vi "Robot Global Data.vi"() -> ()   [LabVIEW 2020]
doc: "This global VI can contain as many global variables as you need. To create a global variable, place a control on the panel, give it a good name. To read or write to it from a VI, drag the icon to the diagram of that VI. You can also drag from the project. Click on the node to change which global you access. You shouldn't have multiple locations writing to a global or it will cause a race-condition."
uses:
  <vilib>/Rock Robotics/WPI/Camera/WPI_CameraImageSize.ctl
  <vilib>/Rock Robotics/WPI/DriverStation/WPI_DriverStationRobotMode2.ctl
  Support Code/submodules/bordeaux-pathinator/Bordeaux/Types/Single Cmd Info.ctl
  <vilib>/picture/picture.llb/imagedata.ctl
  Support Code/submodules/bordeaux-pathinator/Bordeaux/Types/Trajectory Data.ctl
  Support Code/submodules/bordeaux-pathinator/Bordeaux/Types/Segment Type.ctl
  Support Code/submodules/bordeaux-pathinator/Bordeaux/Types/Overrides.ctl
  Support Code/submodules/bordeaux-pathinator/Bordeaux/Types/Angluar Limits.ctl
  Support Code/submodules/bordeaux-pathinator/Bordeaux/Types/Drive Type.ctl
  Support Code/submodules/bordeaux-pathinator/Bordeaux/Types/Path Type.ctl
  Support Code/submodules/numlock/src/numlock.ctl
panel:
  out "Shooter Ready?":bool
  in  "Deadman Switch Active":bool
  out "Climb Sequence Finished":bool
  out "logger":T1
  out "Autos":T10(array[cluster]) {"Fields"."Overrides"."Angle Override" step=5.0; "Fields"."Overrides"."Velocity Override" step=5.0; "Fields"."Overrides"."Angular Override" step=5.0; "Fields"."Angular Limits"."Jerk (deg/s^3)" min=0.0 step=1.0; "Fields"."Angular Limits"."Accel (deg/s^2)" min=0.0; "Fields"."Angular Limits"."Velocity (deg/s)" min=0.0}
  in  "One At a Time":T11={"LF"=TRUE, "LB"=TRUE, "RF"=TRUE, "RB"=TRUE}
  in  "Robot Mode":T12
  in  "image size":T13=enum."320x240"
  in  "Enable Vision":bool
  # "10 12 11 9"
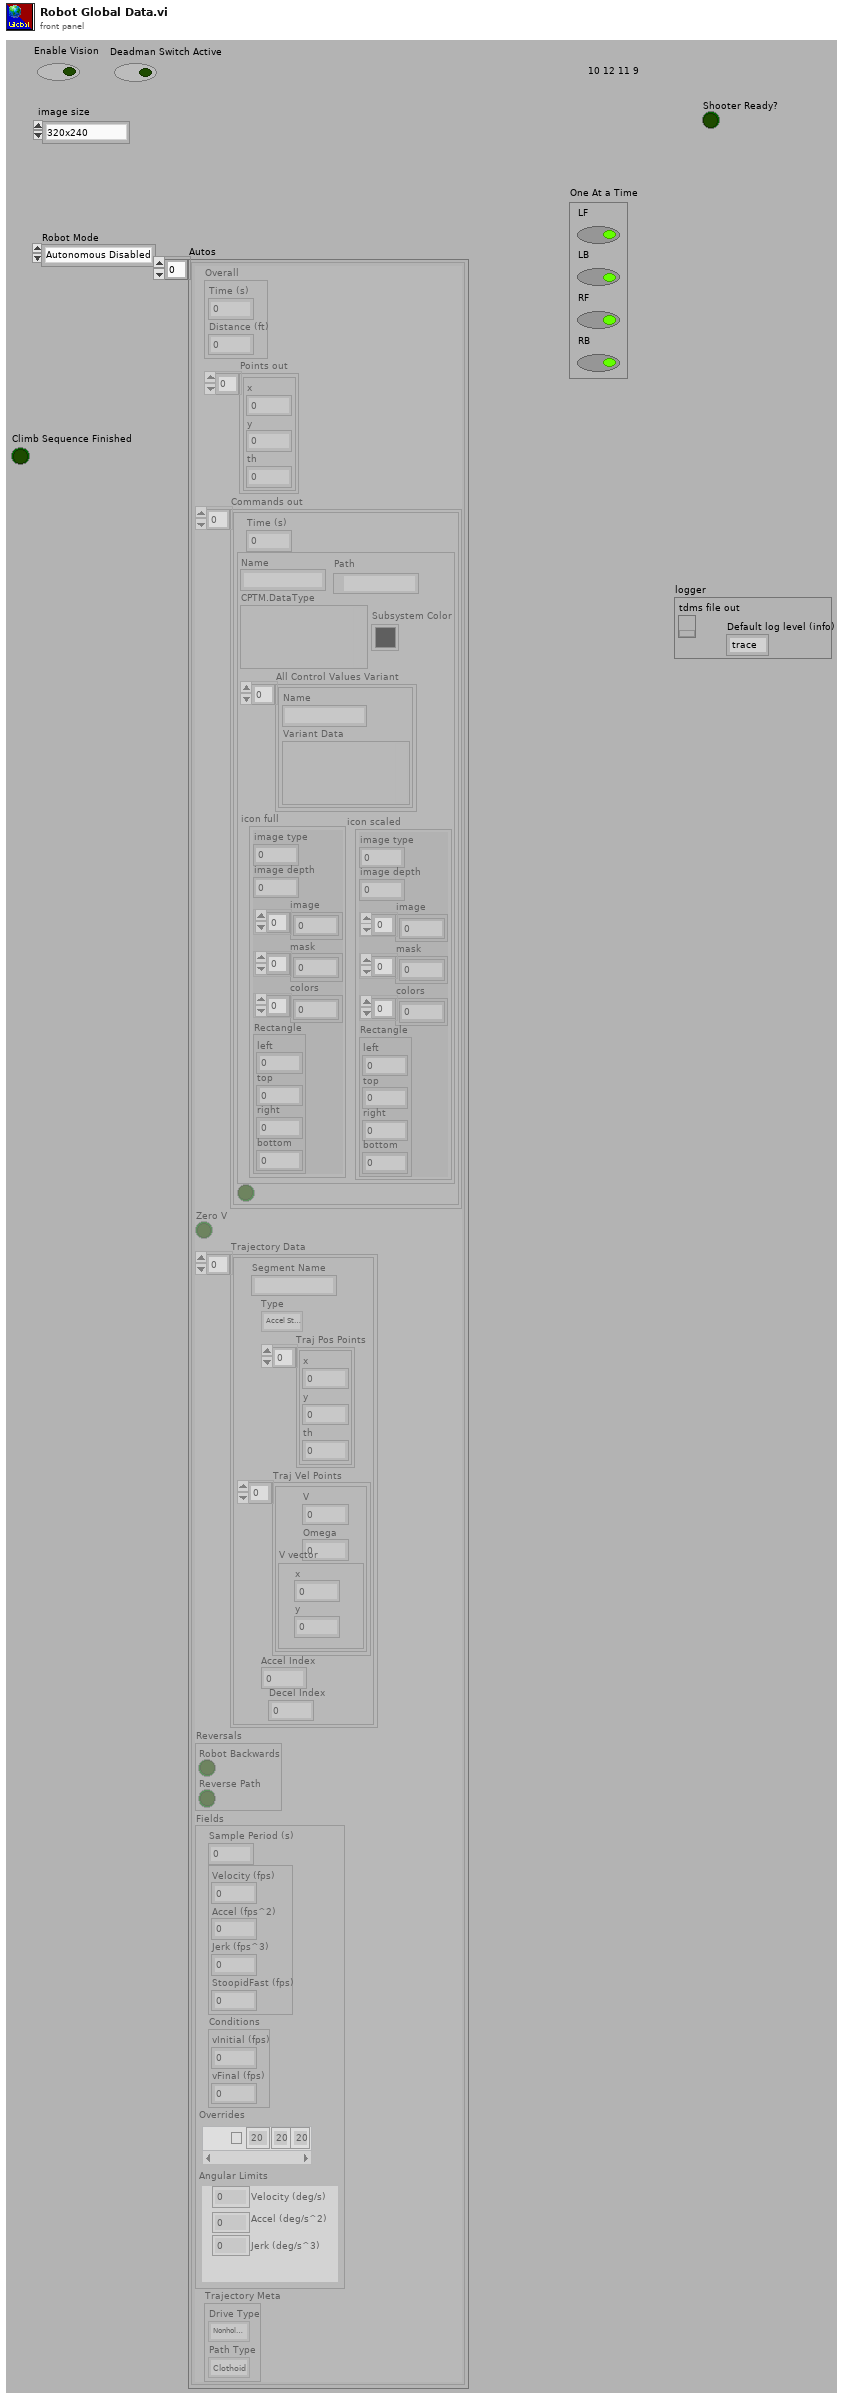
[diagram p1: front panel]
types:
  T1 = typedef "numlock.ctl" = cluster{"tdms file out":refnum<k34>, "Default log level (info)":enum16{"trace", "debug", "info", "warn", "error"}}
  T2 = typedef "Single Cmd Info.ctl" = cluster{"Name":string, "CPTM.DataType":variant, "All Control Values Variant":cluster{"Name":string, "Variant Data":variant}[], "icon full":T3, "icon scaled":T3, "Path":path, "Subsystem Color":u32}
  T3 = typedef "imagedata.ctl" = cluster{"image type":i32, "image depth":i32, "image":u8[], "mask":u8[], "colors":u32[], "Rectangle":cluster{"left":i16, "top":i16, "right":i16, "bottom":i16}}
  T4 = typedef "Trajectory Data.ctl" = cluster{"Segment Name":string, "Type":T5, "Traj Pos Points":cluster{"x":dbl, "y":dbl, "th":dbl}[], "Traj Vel Points":cluster{"V":dbl, "Omega":dbl, "V vector":cluster{"y":dbl, "x":dbl}}[], "Accel Index":i32, "Decel Index":i32}[]
  T5 = typedef "Segment Type.ctl" = enum16{"Accel Straight", "Const Straight", "Blend", "Circle", "Bezier"}
  T6 = typedef "Overrides.ctl" = cluster{"Count":string, "Angular Override":dbl, "Enabled?":bool, "Velocity Override":dbl, "Angle Override":dbl}[]
  T7 = typedef "Angluar Limits.ctl" = cluster{"Velocity (deg/s)":dbl, "Accel (deg/s^2)":dbl, "Jerk (deg/s^3)":dbl}
  T8 = typedef "Drive Type.ctl" = enum16{"Nonholonomic", "Holonomic"}
  T9 = typedef "Path Type.ctl" = enum16{"Clothoid", "Bezier"}
  T10 = cluster{"Overall":cluster{"Time (s)":dbl, "Distance (ft)":dbl}, "Points out":cluster{"x":dbl, "y":dbl, "th":dbl}[], "Commands out":cluster{"Time (s)":dbl, T2, bool}[], "Zero V":bool, "Trajectory Data":T4, "Reversals":cluster{"Robot Backwards":bool, "Reverse Path":bool}, "Fields":cluster{"Sample Period (s)":dbl, cluster{"Velocity (fps)":dbl, "Accel (fps^2)":dbl, "Jerk (fps^3)":dbl, "StoopidFast (fps)":dbl}, "Conditions":cluster{"vInitial (fps)":dbl, "vFinal (fps)":dbl}, "Overrides":T6, "Angular Limits":T7}, "Trajectory Meta":cluster{"Drive Type":T8, "Path Type":T9}}[]
  T11 = cluster{"LF":bool, "LB":bool, "RF":bool, "RB":bool}
  T12 = typedef "WPI_DriverStationRobotMode2.ctl" = enum16{"Autonomous Disabled", "Autonomous Enabled", "Teleop Disabled", "Teleop Enabled", "Disconnected", "Finish", "Test Disabled", "Test Enabled", "Emergency Stopped"}
  T13 = typedef "WPI_CameraImageSize.ctl" = enum16{"640x480", "320x240", "160x120", "Custom"}
diagram:
